vi "Send Msg to MessageLogger.vi"(6 "Severity Code (info)":T1=enum."info", 8 "Error In":errorcluster, 10 "Message Content":string, 11 "Message Tag":string) -> (0 "Error Out":errorcluster)   [LabVIEW 2014, in "CS++Utilities.lvlib"]
doc: "Send mesage to the CS++MessageLogger."
uses:
  CS++Utilities.lvlib
  Base/Severity.ctl
  Classes/CS++BaseClasses/MessageLogger/CS++MessageLogger.lvclass
  Base/CS++Base.lvlib
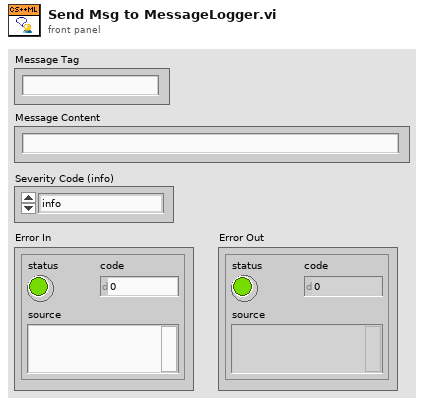
[diagram p1: front panel]
types:
  T1 = typedef "CS++Base.lvlib/Severity.ctl" = enum16{"emergency", "alert", "critical", "error", "warning", "notice", "info", "debug"}
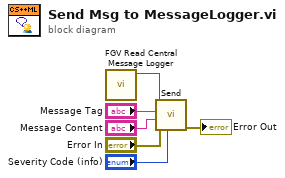
[diagram p0: block diagram]
diagram:
  n1 = call "FGV Read Central Message Logger.vi"() -> ("CS++MessageLogger out"=w6:refnum<class "CS++MessageLogger.lvclass">)  [unwired: 10 in, 1 out]
  n2 = call "Send.vi"("Severity Code (info)"="Severity Code (info)", "Error In"="Error In", "Message Content"="Message Content", "Message Tag"="Message Tag", "CS++MessageLogger in"=w6) -> ("Error Out"=→"Error Out":errorcluster)  [unwired: 5 in, 1 out]
